vi "RenameLib.vi"(0 "LibWriter":refnum<class "LibWriter.lvclass">, 1 "LibRef":refnum<vi>, 2 "NewLibPath":path, 4 "RelinkWholeProject":bool, 5 "error in (no error)":errorcluster) -> (14 "LibWriter":refnum<class "LibWriter.lvclass">, 19 "error out":errorcluster)   [LabVIEW 2014, in "LibWriter.lvclass"]
uses:
  <resource>/Framework/Providers/Open_GDS/ClassProviders/LibProvider_BaseClassInterface/LibWriter_class/ClassWriter_class/LibWriter.lvclass
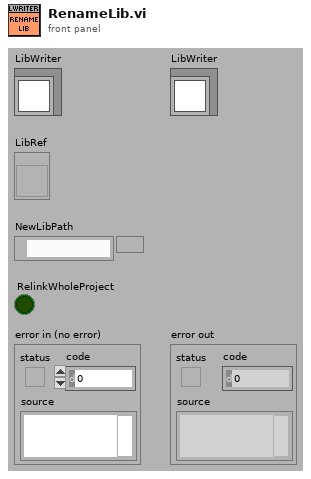
[diagram p1: front panel]
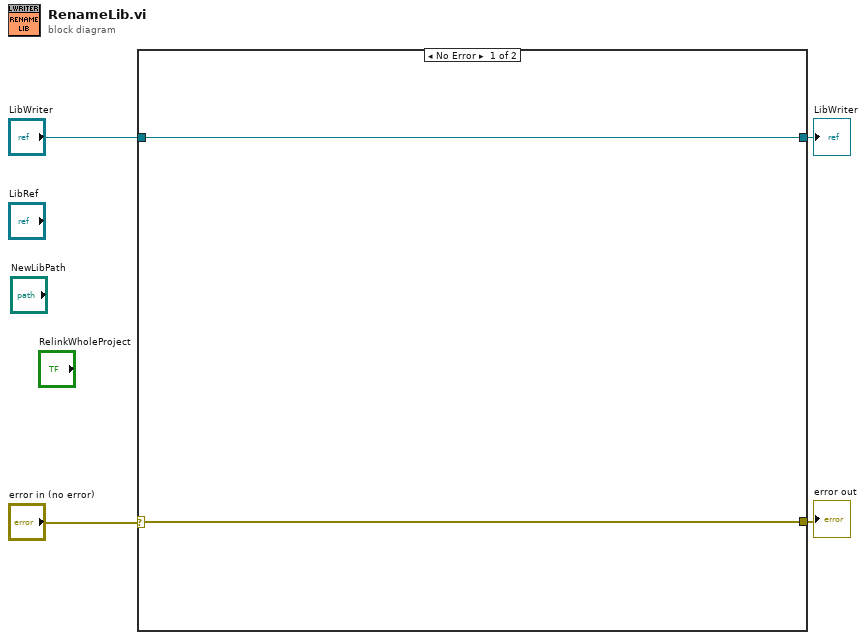
[diagram p0: block diagram]
diagram:
  n1 = case shown="No Error" "error in (no error)" {
    selector: "error in (no error)" -> [w5 w7]
    tunnel: "LibWriter" -> [w6 w8]
    tunnel: [w5 w7] -> w3
    tunnel: [w6 w8] -> w2
    frame No Error {
    }
    frame Error {
    }
  }
  "LibWriter" <- w2
  "error out" <- w3
